vi "曲线对齐 - 副本.vi"() -> ()   [LabVIEW 2015]
uses:
  <vilib>/Utility/miscctls.llb/LVCursorListTypeDef.ctl
  <vilib>/Utility/file.llb/Read Delimited Spreadsheet (DBL).vi
panel:
  in  "确认修改":bool
  in  "功能选择":enum16{"无", "缩放实际曲线", "缩放理论曲线"}(ring)
  in  "加载数据":bool
  out "XY图 3":cluster{"理论时间":dbl[], "力":dbl[]}[](graph)
  out "all rows 2":dbl[][](array[numeric]) caption="所有行"
  in  "理论曲线路径":path=path "D:/曲线处理/理论1.csv" caption="理论"
  out "all rows":dbl[][](array[numeric]) caption="所有行"
  in  "测量曲线路径":path=path "D:/曲线处理/实测1.csv" caption="实际"
  in  "Enqueue Element":bool caption="元素入队列"
  in  "时间缩放 2":dbl=1.0
  in  "确定移动":bool
  out "输出簇 4":cluster{"x":dbl[], "y":dbl[]}
  out "输出簇 3":cluster{"x":dbl[], "y":dbl[]}
  out "输出簇 2":cluster{"x":dbl[], "y":dbl[]}
  out "输出簇1":cluster{"x":dbl[], "y":dbl[]}
  out "XY图 2":cluster{"x":dbl[], "y":dbl[]}[](graph)
  out "Position.X":dbl
  out "min(x,y)":dbl
  out "max(x,y)":dbl
  out "游标位置":cluster{"X":dbl, "Y":dbl}
  in  "动作":enum16{"设置范围", "设置峰值", "移动峰值"}(ring)
  in  "停止":bool
  in  "max":dbl=12.0 format="%#_13g"
  in  "min":dbl
  in  "力偏移":dbl
  in  "力缩放":dbl=1.0
  in  "时间偏移":dbl
  in  "时间缩放":dbl=1.0
  out "XY图":cluster{dbl[], dbl[]}[](graph)
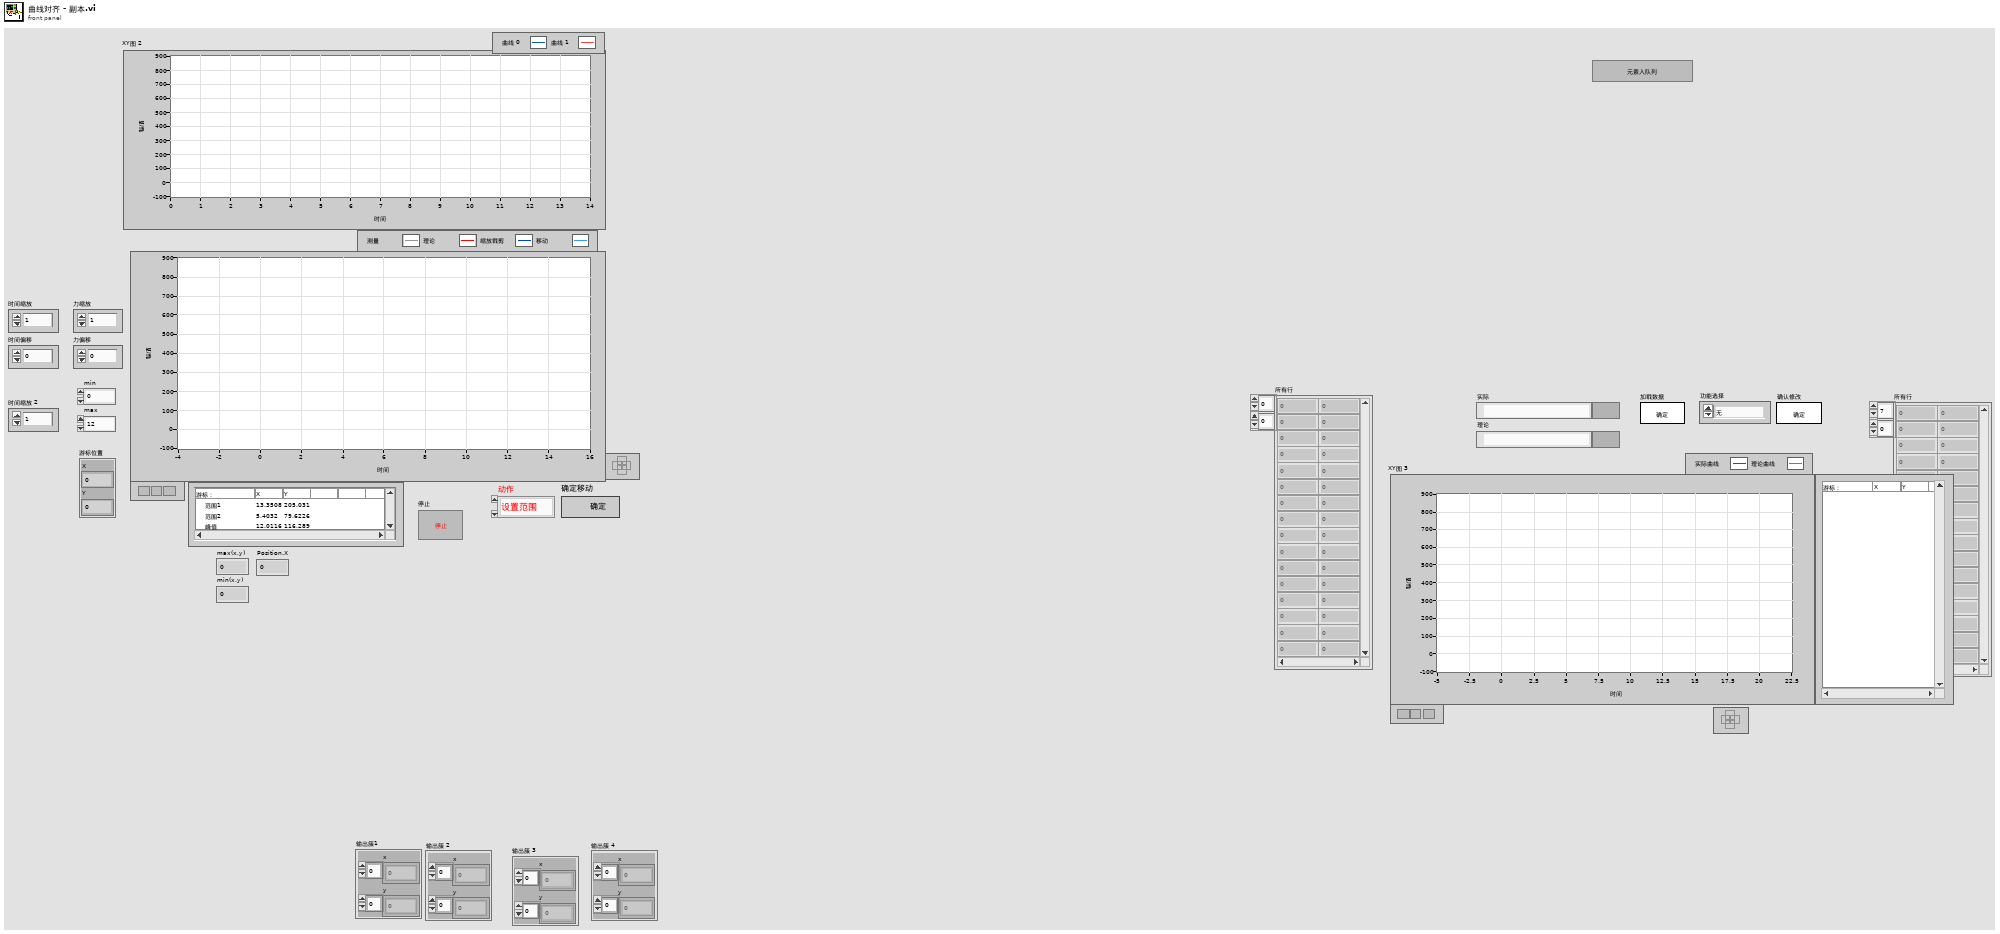
[diagram p1: front panel]
types:
  T1 = typedef "LVCursorListTypeDef.ctl" = cluster{"Name":string, "Color":u32, "Style":u8, "Point Style":u8, "Name Visible":bool, "Allow Drag":bool, "Cursor Mode":u32, "Plot":i32, "Index":i32, "Position":cluster{"X":dbl, "Y":dbl}, "X Scale":u32, "Y Scale":u32, "Watch Plots":i32[], "Watch All Plots":bool, "Plot Area":i32, "Label Offset":cluster{"X":dbl, "Y":dbl}}[]
  T2 = cluster{"Name":string, "Color":u32, "Style":u8, "Point Style":u8, "Name Visible":bool, "Allow Drag":bool, "Cursor Mode":u32, "Plot":i32, "Index":i32, "Position":cluster{"X":dbl, "Y":dbl}, "X Scale":u32, "Y Scale":u32, "Watch Plots":i32[], "Watch All Plots":bool, "Plot Area":i32, "Label Offset":cluster{"X":dbl, "Y":dbl}}
  T3 = cluster{"力":dbl[], "时间":dbl[], "理论力":dbl[], "理论时间":dbl[], "力预览":dbl[], "时间预览":dbl[]}
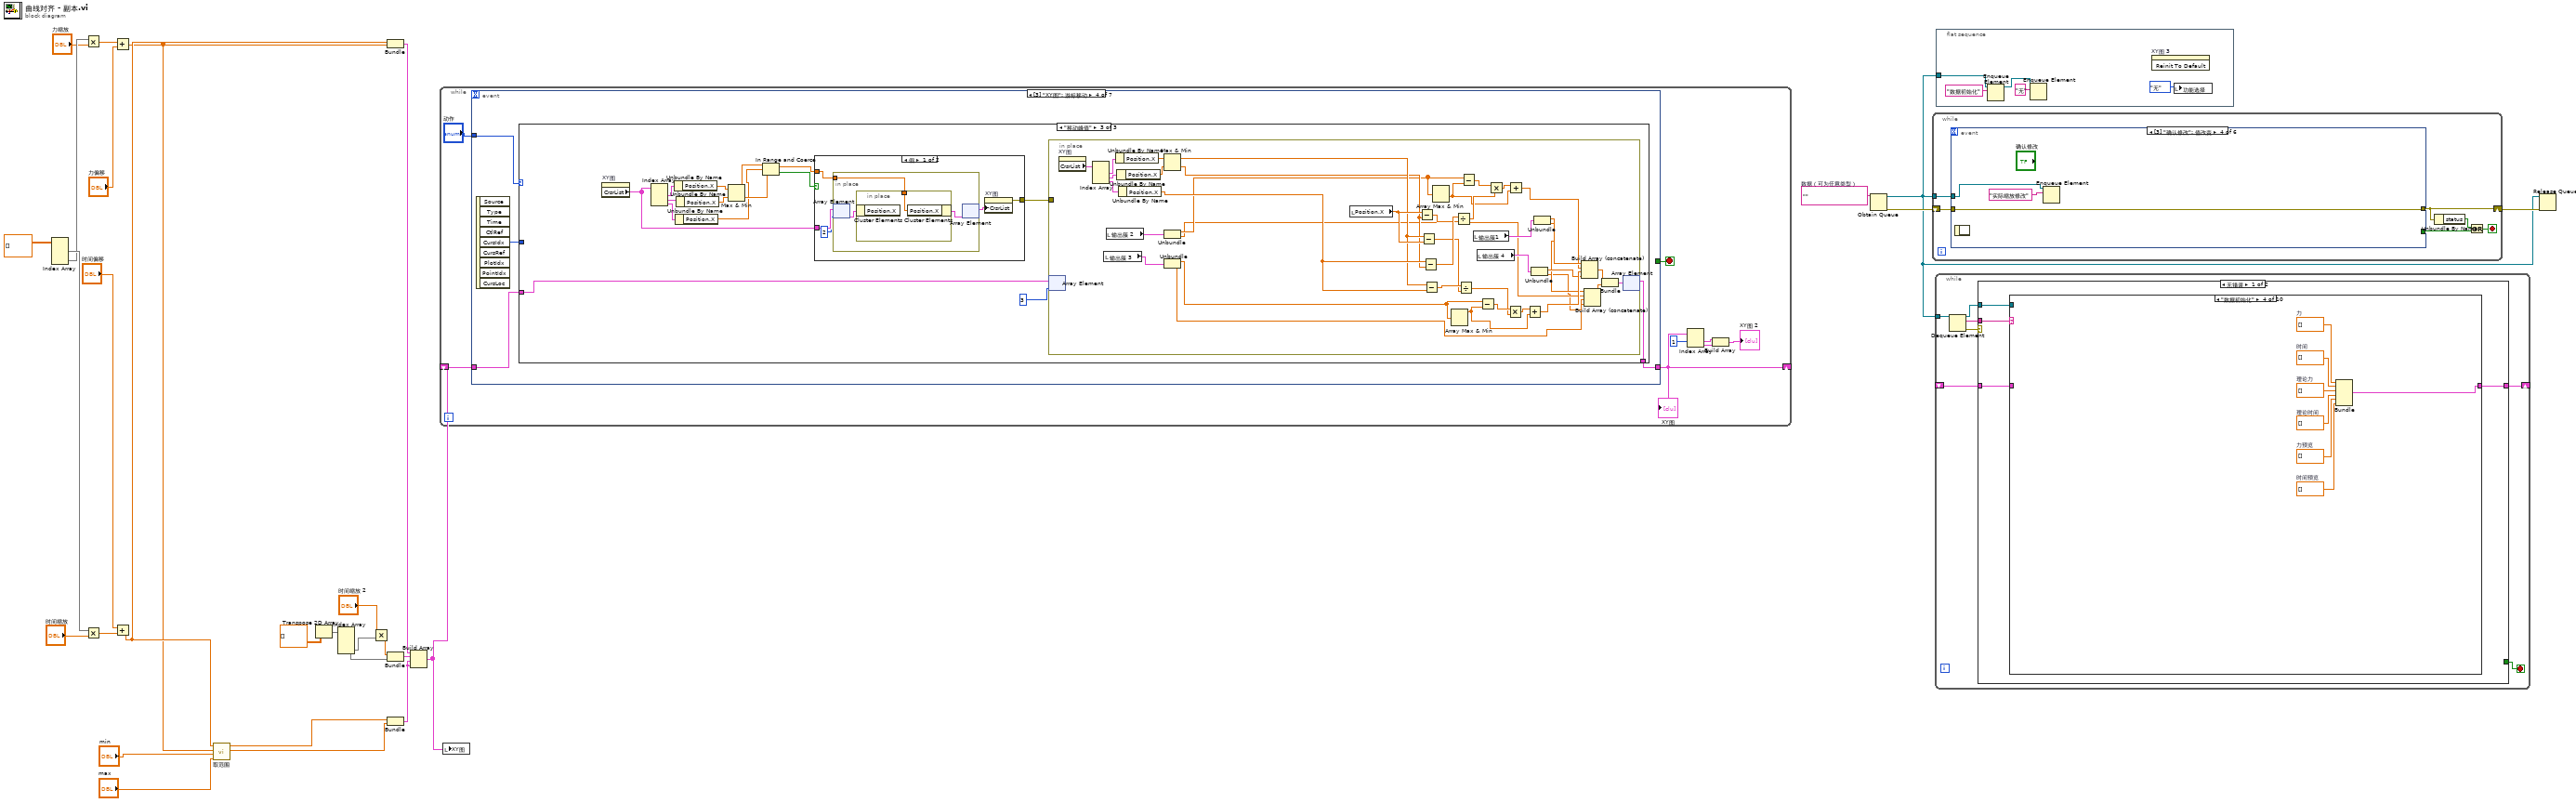
[diagram p0: block diagram]
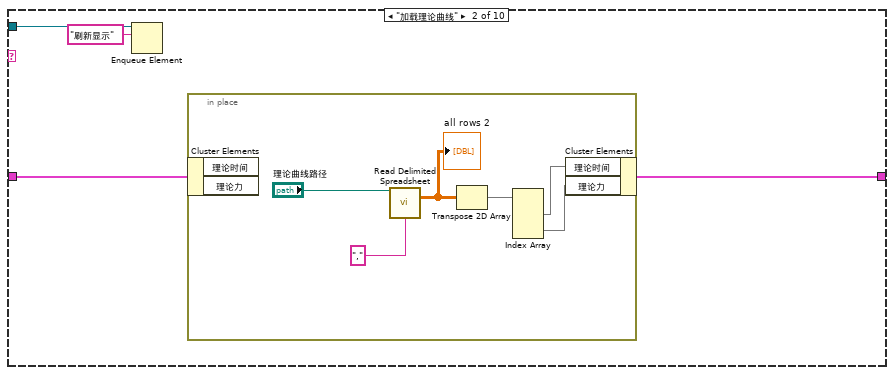
[diagram p3: hidden frame]
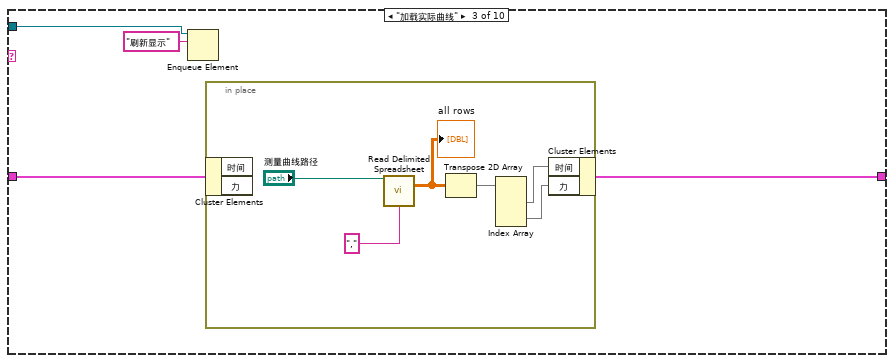
[diagram p4: hidden frame]
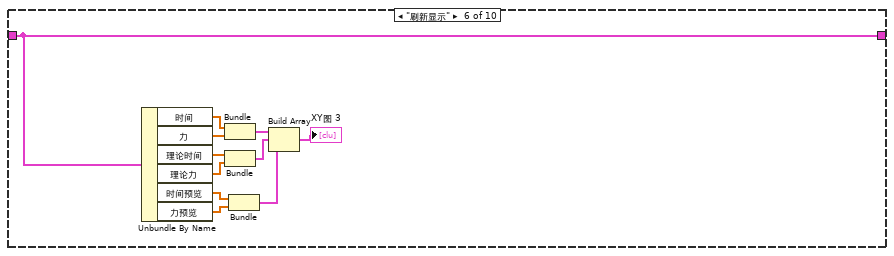
[diagram p6: hidden frame]
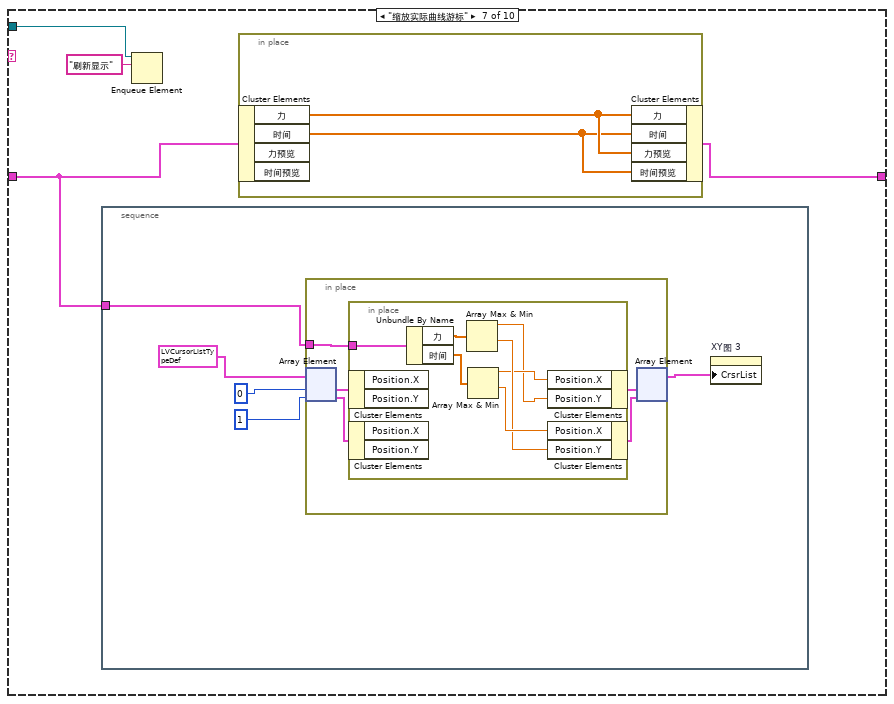
[diagram p7: hidden frame]
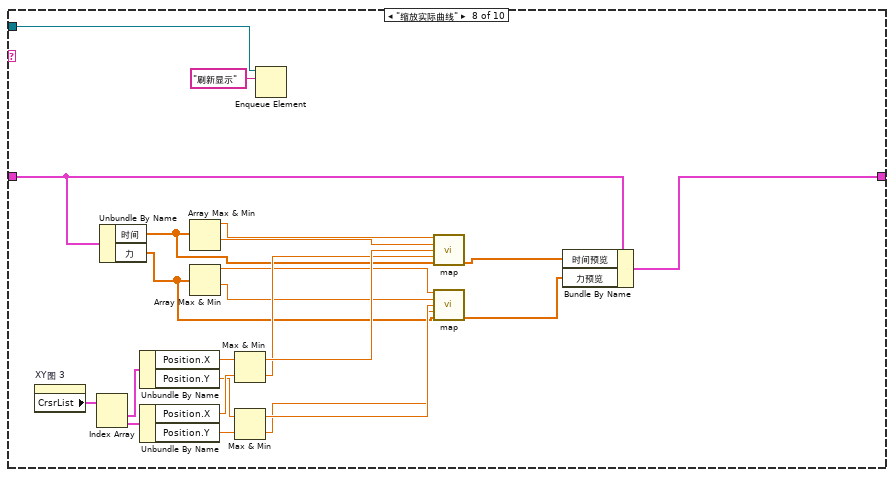
[diagram p8: hidden frame]
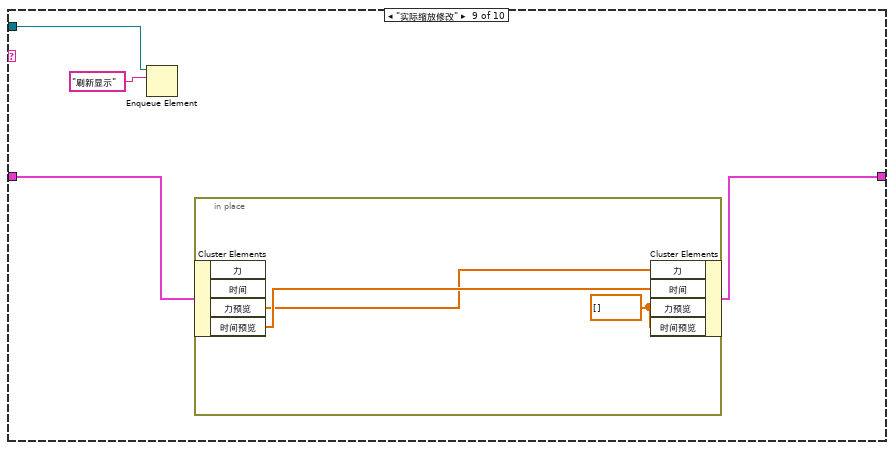
[diagram p9: hidden frame]
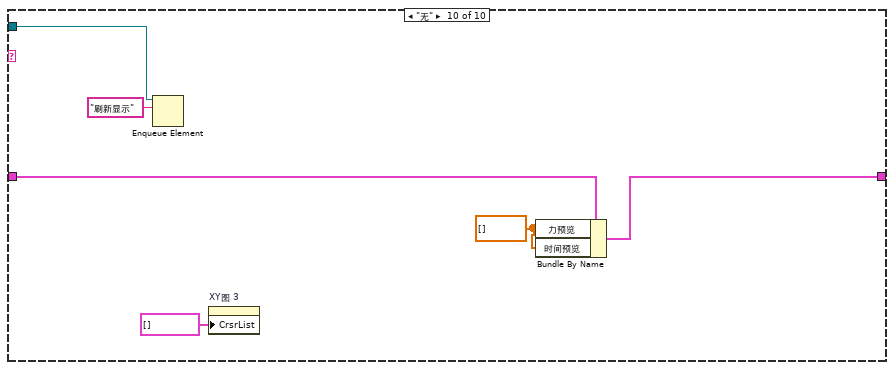
[diagram p10: hidden frame]
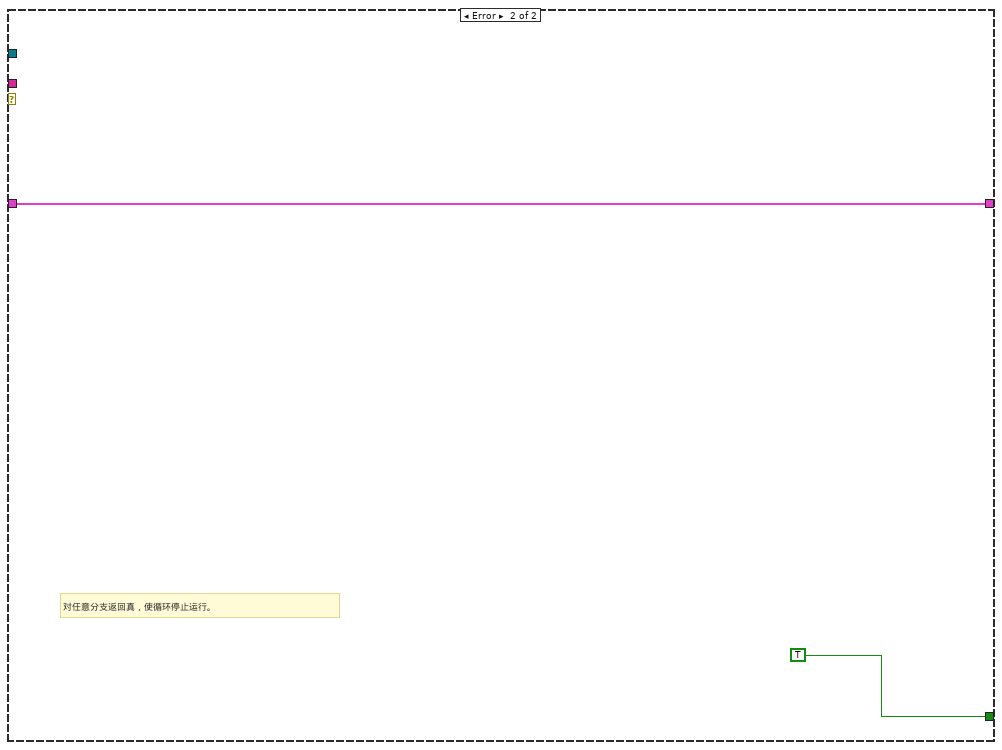
[diagram p11: hidden frame]
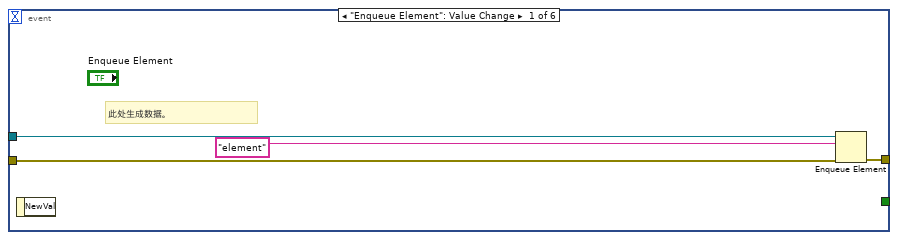
[diagram p12: hidden frame]
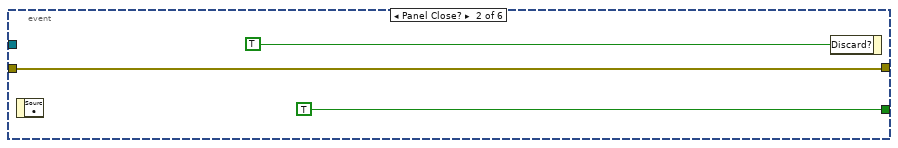
[diagram p13: hidden frame]
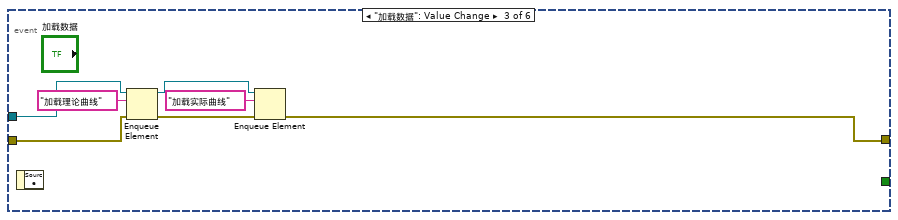
[diagram p14: hidden frame]
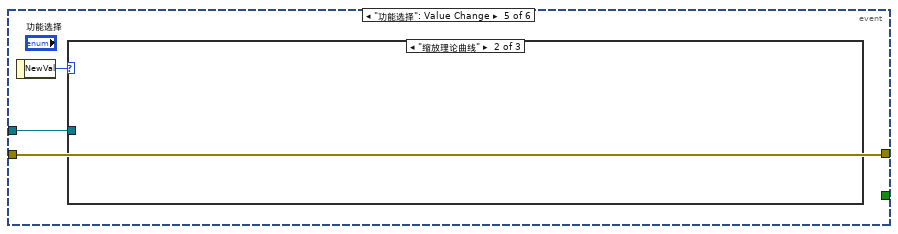
[diagram p15: hidden frame]
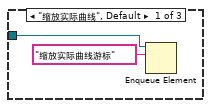
[diagram p16: hidden frame]
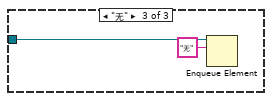
[diagram p17: hidden frame]
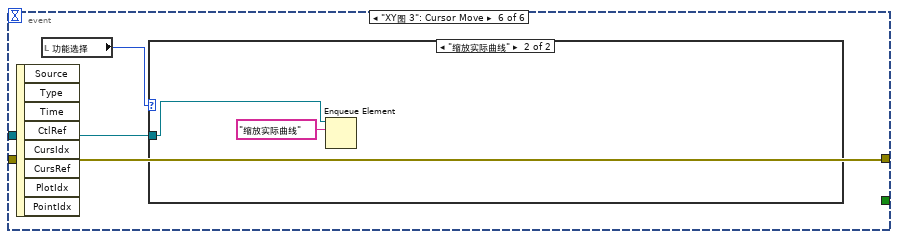
[diagram p18: hidden frame]
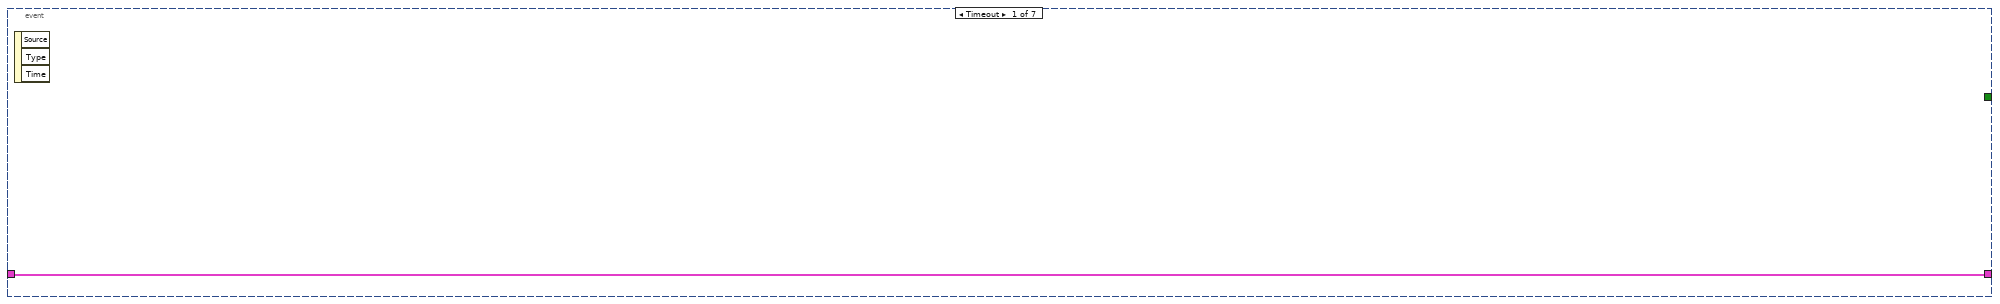
[diagram p20: hidden frame]
diagram:
  w6 = ""  # 数据（可为任意类型）
  n1 = Index Array(array=dbl[][] [] ("转置的数组")) -> (element #1=w25:dbl[], element #2=w21:dbl[])  [unwired: 4 in]
  n2 = Multiply(x=w21, y="力缩放") -> (x*y=w18:dbl[])
  n3 = Multiply(x=w25, y="时间缩放") -> (x*y=w22:dbl[])
  n4 = Add(x=w18, y="力偏移") -> (x+y=w12:dbl[])
  n5 = Add(x="时间偏移", y=w22) -> (x+y=w13:dbl[])
  n6 = call "取范围.vi"("max"="max", "min"="min", "y"=w12, "x"=w13) -> ("y"=w16:dbl[], "x"=w17:dbl[])  [unwired: 6 in]
  n7 = Transpose 2D Array(2D array=dbl[][] [] ("all rows")) -> (transposed array=w28:dbl[][])
  n8 = Index Array(array=w28) -> (element #1=w8:dbl[], element #2=w29:dbl[])  [unwired: 4 in]
  n9 = Multiply(x="时间缩放 2", y=w8) -> (x*y=w7:dbl[])
  n10 = Bundle(w13, w12) -> (w26:cluster{dbl[], dbl[]})  [unwired: 1 in]
  n11 = Bundle(w7, w29) -> (w27:cluster{dbl[], dbl[]})  [unwired: 1 in]
  n12 = Bundle("x"=w17, "y"=w16) -> (w11:cluster{"x":dbl[], "y":dbl[]})  [unwired: 1 in]
  n13 = Build Array(w26, w27, w11, w11) -> (w10:cluster{"x":dbl[], "y":dbl[]}[])
  n14 = while {
    shift-right: [w34] -> _
    shift-left: w10 -> [w35]
    stop <- w37 stop-if-true
    n15 = event shown="[3] \"XY图\": 游标移动" {
      selector: _ -> [_ _ _ _ _ _ _]
      dyn-events: _ -> [_ _ _ _ _ _ _]
      timeout: _ -> [_ _ _ _ _ _ _]
      tunnel: [_ _ _ _ _ _ TRUE] -> w37
      tunnel: "动作" -> [_ w40 w54 w66 _ _ _]
      tunnel: w35 -> [w38 w39 w53 w64 w163 w166 w211]
      tunnel: [w38 w39 w53 w63 w162 w166 w211] -> w34
      event Timeout {
        n16 = event-data() -> ()  [unwired: 1 in, 3 out]
      }
      event "XY图": event type 3.0.x80000027 {
        n17 = event-data() -> ("CursIdx"=w42:i32)  [unwired: 1 in, 7 out]
        n18 = case shown="\"设置峰值\"" w40 {
          tunnel: w42 -> [w45 w48 w51]
          tunnel: [w43 w46 w49] -> w41
          frame "设置范围", Default {
            n19 = Equal?(x=w45, y=2) -> (x = y?=w43:bool)
          }
          frame "设置峰值" {
            n20 = Not Equal?(x=w48, y=2) -> (x != y?=w46:bool)
          }
          frame "移动峰值" {
            n21 = Not Equal?(x=w51, y=2) -> (x != y?=w49:bool)
          }
        }
        n22 = event-data("Discard?"=w41) -> ()  [unwired: 1 in, 1 out]
      }
      event "XY图": Cursor Release {
        n23 = event-data() -> ("CursLoc"=→"游标位置":cluster{"X":dbl, "Y":dbl})  [unwired: 1 in, 8 out]
        n24 = property on="XY图" class="XYGraph (严格)"() -> ("CrsrList"=w52:T1)  [unwired: 2 in, 2 out]
        n25 = case shown="\"设置范围\", 默认" w54 {
          tunnel: w52 -> [w56 _ _]
          frame "设置范围", Default {
            n26 = Index Array(array=w56) -> (element #1=w62:T2, element #2=w61:T2)  [unwired: 2 in]
            n27 = Unbundle By Name(w62) -> ("Position.X"=w60:dbl)
            n28 = Unbundle By Name(w61) -> ("Position.X"=w59:dbl)
            n29 = Max & Min(x=w60, y=w59) -> (max(x,y)=→"max(x,y)":dbl, min(x,y)=→"min(x,y)":dbl)
          }
          frame "设置峰值" {
          }
          frame "移动峰值" {
          }
        }
      }
      event "XY图": Cursor Move {
        n30 = event-data() -> ("CursIdx"=w65:i32)  [unwired: 1 in, 8 out]
        n31 = case shown="\"移动峰值\"" w66 {
          tunnel: w65 -> [_ w76 _]
          tunnel: w64 -> [w67 w68 w112]
          tunnel: [w67 w68 w98] -> w63
          frame "设置范围", Default {
          }
          frame "设置峰值" {
            n32 = Equal?(x=w76, y=2) -> (x = y?=w74:bool)
            n33 = case shown="真" w74 {
              tunnel: [_ w77] -> w69
              frame False {
              }
              frame True {
                n34 = property on="XY图" class="XYGraph (严格)"() -> ("CrsrList"=w78:T1)  [unwired: 2 in, 2 out]
                n35 = Index Array(array=w78) -> (element #1=w87:T2, element #2=w86:T2, element #3=w88:T2)  [unwired: 3 in]
                n36 = Unbundle By Name(w87) -> ("Position.X"=w85:dbl)
                n37 = Unbundle By Name(w88) -> ("Position.X"=w81:dbl)
                n38 = Unbundle By Name(w86) -> ("Position.X"=w84:dbl)
                n39 = Max & Min(x=w85, y=w84) -> (max(x,y)=w83:dbl, min(x,y)=w82:dbl)
                n40 = In Range and Coerce(upper limit=w83, x=w81, lower limit=w82) -> (coerced(x)=w79:dbl, In Range?=w80:bool)
                n41 = case shown="假" w80 {
                  tunnel: w79 -> [w91 _]
                  tunnel: w78 -> [w93 _]
                  tunnel: [w89 _] -> w77
                  frame False {
                    n42 = in-place {
                      in-place-border: w91 -> [w95]
                      n43 = in-place-array #1(w93, 2) -> (w96:T2)
                      n44 = in-place {
                        in-place-border: w95 -> [w97]
                        n45 = in-place-cluster #2(w96) -> ()  [unwired: 1 out]
                        n46 = in-place-cluster #2("Position.X"=w97) -> (w94:T2)
                      }
                      n47 = in-place-array #1(w94) -> (w90:T1)  [unwired: 1 out]
                    }
                    n48 = property on="XY图" class="XYGraph (严格)"("CrsrList"=w90) -> (error out=w89:errorcluster)  [unwired: 2 in, 1 out]
                  }
                  frame True {
                  }
                }
              }
            }
            n49 = property on="XY图" class="XYGraph (严格)"(error in=w69) -> ("CrsrList"=w73:T1)  [unwired: 1 in, 2 out]
            n50 = Index Array(array=w73, index=2 ("索引")) -> (element=w71:T2)
            n51 = Unbundle By Name(w71) -> ("Position.X"=→"Position.X":dbl)
          }
          frame "移动峰值" {
            n52 = property on="XY图" class="XYGraph (严格)"() -> ("CrsrList"=w100:T1)  [unwired: 2 in, 2 out]
            n53 = Index Array(array=w100) -> (element #1=w109:T2, element #2=w108:T2, element #3=w110:T2)  [unwired: 3 in]
            n54 = Unbundle By Name(w109) -> ("Position.X"=w107:dbl)
            n55 = Unbundle By Name(w110) -> ("Position.X"=w103:dbl)
            n56 = Unbundle By Name(w108) -> ("Position.X"=w106:dbl)
            n57 = Max & Min(x=w107, y=w106) -> (max(x,y)=w105:dbl, min(x,y)=w104:dbl)
            n58 = In Range and Coerce(upper limit=w105, x=w103, lower limit=w104) -> (coerced(x)=w101:dbl, In Range?=w102:bool)
            n59 = case shown="假" w102 {
              tunnel: w101 -> [w115 _]
              tunnel: w100 -> [w117 _]
              tunnel: [w113 _] -> w99
              frame False {
                n60 = in-place {
                  in-place-border: w115 -> [w119]
                  n61 = in-place-array #3(w117, 2) -> (w120:T2)
                  n62 = in-place {
                    in-place-border: w119 -> [w121]
                    n63 = in-place-cluster #4(w120) -> ()  [unwired: 1 out]
                    n64 = in-place-cluster #4("Position.X"=w121) -> (w118:T2)
                  }
                  n65 = in-place-array #3(w118) -> (w114:T1)  [unwired: 1 out]
                }
                n66 = property on="XY图" class="XYGraph (严格)"("CrsrList"=w114) -> (error out=w113:errorcluster)  [unwired: 2 in, 1 out]
              }
              frame True {
              }
            }
            n67 = in-place {
              in-place-border: w99 -> [_]
              n68 = in-place-array #5(w112, 3) -> ()  [unwired: 1 out]
              n69 = property on="XY图" class="XYGraph (严格)"() -> ("CrsrList"=w160:T1)  [unwired: 2 in, 2 out]
              n70 = Index Array(array=w160) -> (element #1=w159:T2, element #2=w158:T2, element #3=w155:T2)  [unwired: 3 in]
              n71 = local read "输出簇 3"() -> (w138:cluster{"x":dbl[], "y":dbl[]})
              n72 = local read "输出簇 2"() -> (w139:cluster{"x":dbl[], "y":dbl[]})
              n73 = Unbundle By Name(w159) -> ("Position.X"=w157:dbl)
              n74 = Unbundle By Name(w158) -> ("Position.X"=w156:dbl)
              n75 = Unbundle By Name(w155) -> ("Position.X"=w153:dbl)
              n76 = Unbundle(w139) -> ("x"=w137:dbl[], "y"=w127:dbl[])
              n77 = Unbundle(w138) -> ("x"=w136:dbl[], "y"=w122:dbl[])
              n78 = Max & Min(x=w157, y=w156) -> (max(x,y)=w152:dbl, min(x,y)=w151:dbl)
              n79 = local read "Position.X"() -> (w154:dbl)
              n80 = Subtract(x=w154, y=w151) -> (x-y=w149:dbl)
              n81 = Subtract(x=w152, y=w154) -> (x-y=w147:dbl)
              n82 = Subtract(x=w153, y=w151) -> (x-y=w150:dbl)
              n83 = Subtract(x=w152, y=w153) -> (x-y=w148:dbl)
              n84 = Array Max & Min(array=w137) -> (min value=w143:dbl)  [unwired: 3 out]
              n85 = Array Max & Min(array=w136) -> (max value=w135:dbl)  [unwired: 3 out]
              n86 = Divide(x=w150, y=w149) -> (x/y=w145:dbl)
              n87 = Divide(x=w148, y=w147) -> (x/y=w140:dbl)
              n88 = Subtract(x=w137, y=w143) -> (x-y=w146:dbl[])
              n89 = local read "输出簇1"() -> (w134:cluster{"x":dbl[], "y":dbl[]})
              n90 = local read "输出簇 4"() -> (w133:cluster{"x":dbl[], "y":dbl[]})
              n91 = Subtract(x=w136, y=w135) -> (x-y=w141:dbl[])
              n92 = Multiply(x=w146, y=w145) -> (x*y=w144:dbl[])
              n93 = Multiply(x=w141, y=w140) -> (x*y=w142:dbl[])
              n94 = Add(x=w144, y=w143) -> (x+y=w131:dbl[])
              n95 = Add(x=w142, y=w135) -> (x+y=w130:dbl[])
              n96 = Unbundle(w133) -> ("x"=w129:dbl[], "y"=w126:dbl[])
              n97 = Unbundle(w134) -> ("x"=w132:dbl[], "y"=w128:dbl[])
              n98 = Build Array (concatenate)(w132, w131, w130, w129) -> (w125:dbl[])
              n99 = Build Array (concatenate)(w128, w127, w122, w126) -> (w124:dbl[])
              n100 = Bundle(w125, w124) -> (w123:cluster{dbl[], dbl[]})  [unwired: 1 in]
              n101 = in-place-array #5(w123) -> (w98:cluster{"x":dbl[], "y":dbl[]}[])  [unwired: 1 out]
            }
          }
        }
      }
      event "确定移动": Value Change {
        n102 = event-data() -> ()  [unwired: 1 in, 6 out]
        n103 = in-place {
          n104 = in-place-array #6(w163, 2, 3) -> (w165:cluster{"x":dbl[], "y":dbl[]})  [unwired: 1 out]
          n105 = in-place-array #6(w165, w165) -> (w162:cluster{"x":dbl[], "y":dbl[]}[])  [unwired: 2 out]
        }
      }
      event "动作": Value Change {
        n106 = event-data() -> ("NewVal"=w167:enum16{"设置范围", "设置峰值", "移动峰值"})  [unwired: 1 in, 5 out]
        n107 = case shown="\"设置峰值\"" w167 {
          tunnel: w166 -> [_ _ w189]
          frame "设置范围", Default {
          }
          frame "设置峰值" {
            n108 = case shown="真" TRUE {
              frame False {
              }
              frame True {
                n109 = property on="XY图" class="XYGraph (严格)"() -> ("CrsrList"=w176:T1)  [unwired: 2 in, 2 out]
                n110 = Index Array(array=w176) -> (element #1=w178:T2, element #2=w177:T2)  [unwired: 2 in]
                n111 = Unbundle By Name(w178) -> ("Position.X"=w175:dbl)
                n112 = Unbundle By Name(w177) -> ("Position.X"=w174:dbl)
                n113 = Add(x=w175, y=w174) -> (x+y=w173:dbl)
                n114 = Divide(x=w173, y=2.0) -> (x/y=w169:dbl)
                n115 = local write "Position.X"(w169) -> ()
                n116 = in-place {
                  in-place-border: w169 -> [w179]
                  n117 = in-place-array #7(w176, 2) -> (w181:T2)
                  n118 = in-place {
                    in-place-border: w179 -> [w182]
                    n119 = in-place-cluster #8(w181) -> ()  [unwired: 1 out]
                    n120 = in-place-cluster #8("Position.X"=w182) -> (w180:T2)
                  }
                  n121 = in-place-array #7(w180) -> (w170:T1)  [unwired: 1 out]
                }
                n122 = property on="XY图" class="XYGraph (严格)"("CrsrList"=w170) -> ()  [unwired: 2 in, 2 out]
              }
            }
          }
          frame "移动峰值" {
            n123 = Index Array(array=w189, index=2 ("索引")) -> (element=w187:cluster{"x":dbl[], "y":dbl[]})
            n124 = property on="XY图" class="XYGraph (严格)"() -> ("CrsrList"=w210:T1)  [unwired: 2 in, 2 out]
            n125 = Unbundle(w187) -> ("x"=w203:dbl[], "y"=w202:dbl[])
            n126 = Index Array(array=w210) -> (element #1=w209:T2, element #2=w208:T2, element #3=w205:T2)  [unwired: 3 in]
            n127 = Array Max & Min(array=w203) -> (max value=w201:dbl, min value=w204:dbl)  [unwired: 2 out]
            n128 = Unbundle By Name(w209) -> ("Position.X"=w207:dbl)
            n129 = Unbundle By Name(w208) -> ("Position.X"=w206:dbl)
            n130 = Unbundle By Name(w205) -> ("Position.X"=w196:dbl)
            n131 = Max & Min(x=w207, y=w206) -> (max(x,y)=w195:dbl, min(x,y)=w194:dbl)
            n132 = call "取范围.vi"("max"=w194, "min"=w204, "y"=w202, "x"=w203) -> ("y"=w199:dbl[], "x"=w200:dbl[])  [unwired: 6 in]
            n133 = call "取范围.vi"("max"=w196, "min"=w194, "y"=w202, "x"=w203) -> ("y"=w190:dbl[], "x"=w193:dbl[])  [unwired: 6 in]
            n134 = call "取范围.vi"("max"=w195, "min"=w196, "y"=w202, "x"=w203) -> ("y"=w191:dbl[], "x"=w192:dbl[])  [unwired: 6 in]
            n135 = call "取范围.vi"("max"=w201, "min"=w195, "y"=w202, "x"=w203) -> ("y"=w197:dbl[], "x"=w198:dbl[])  [unwired: 6 in]
            n136 = Bundle("x"=w200, "y"=w199) -> (→"输出簇1":cluster{"x":dbl[], "y":dbl[]})  [unwired: 1 in]
            n137 = Bundle("x"=w192, "y"=w191) -> (→"输出簇 3":cluster{"x":dbl[], "y":dbl[]})  [unwired: 1 in]
            n138 = Bundle("x"=w198, "y"=w197) -> (→"输出簇 4":cluster{"x":dbl[], "y":dbl[]})  [unwired: 1 in]
            n139 = Bundle("x"=w193, "y"=w190) -> (→"输出簇 2":cluster{"x":dbl[], "y":dbl[]})  [unwired: 1 in]
          }
        }
      }
      event "停止": Value Change {
        n140 = event-data() -> ()  [unwired: 1 in, 6 out]
      }
    }
    "XY图" <- w34
    n141 = Index Array(array=w34, index #1=1 ("索引")) -> (element #1=w32:cluster{"x":dbl[], "y":dbl[]}, element #2=w31:cluster{"x":dbl[], "y":dbl[]})  [unwired: 1 in]
    n142 = Build Array(w32, w31) -> (→"XY图 2":cluster{"x":dbl[], "y":dbl[]}[])
  }
  n143 = local write "XY图"(w10) -> ()
  n144 = Obtain Queue(element data type=w6) -> (queue out=w1:refnum<queue>, error out=w4:errorcluster)  [unwired: 4 in, 1 out]
  n145 = while {
    shift-right: [w214] -> w5
    shift-left: w4 -> [w217]
    tunnel: w1 -> [w218]
    stop <- w215 stop-if-true
    n146 = event shown="[3] \"确认修改\": 值改变" {
      selector: _ -> [_ _ _ _ _ _]
      dyn-events: _ -> [_ _ _ _ _ _]
      timeout: _ -> [_ _ _ _ _ _]
      tunnel: w218 -> [w222 _ w230 w233 w236 w243]
      tunnel: w217 -> [w221 w225 w227 w235 w238 w245]
      tunnel: [w220 w225 w226 w235 w238 w245] -> w214
      tunnel: [_ TRUE ("stop") _ _ _ _] -> w216
      event "Enqueue Element": Value Change {
        # "此处生成数据。"
        n147 = event-data() -> ()  [unwired: 1 in, 1 out]
        n148 = Enqueue Element(queue=w222, element="element", error in (no error)=w221) -> (error out=w220:errorcluster)  [unwired: 1 in, 2 out]
      }
      event Panel Close? {
        n149 = event-data() -> ()  [unwired: 1 in, 1 out]
        n150 = event-data("Discard?"=TRUE ("放弃？")) -> ()  [unwired: 1 in, 1 out]
      }
      event "加载数据": Value Change {
        n151 = event-data() -> ()  [unwired: 1 in, 1 out]
        n152 = Enqueue Element(queue=w230, element="加载理论曲线" ("元素"), error in (no error)=w227) -> (queue out=w229:refnum<queue>, error out=w228:errorcluster)  [unwired: 1 in, 1 out]
        n153 = Enqueue Element(queue=w229, element="加载实际曲线" ("元素"), error in (no error)=w228) -> (error out=w226:errorcluster)  [unwired: 1 in, 2 out]
      }
      event "确认修改": Value Change {
        n154 = event-data() -> ()  [unwired: 1 in, 1 out]
        n155 = Enqueue Element(queue=w233, element="实际缩放修改" ("元素")) -> ()  [unwired: 2 in, 3 out]
      }
      event "功能选择": Value Change {
        n156 = event-data() -> ("NewVal"=w237:enum16{"无", "缩放实际曲线", "缩放理论曲线"})  [unwired: 1 in]
        n157 = case shown="\"缩放理论曲线\"" w237 {
          tunnel: w236 -> [w239 _ w242]
          frame "缩放实际曲线", Default {
            n158 = Enqueue Element(queue=w239, element="缩放实际曲线游标" ("元素")) -> ()  [unwired: 2 in, 3 out]
          }
          frame "缩放理论曲线" {
          }
          frame "无" {
            n159 = Enqueue Element(queue=w242, element="无" ("元素")) -> ()  [unwired: 2 in, 3 out]
          }
        }
      }
      event "XY图 3": Cursor Move {
        n160 = event-data() -> ()  [unwired: 1 in, 8 out]
        n161 = local read "功能选择"() -> (w244:enum16{"无", "缩放实际曲线", "缩放理论曲线"})
        n162 = case shown="\"缩放实际曲线\"" w244 {
          tunnel: w243 -> [_ w246]
          frame "无", Default {
          }
          frame "缩放实际曲线" {
            n163 = Enqueue Element(queue=w246, element="缩放实际曲线" ("元素")) -> ()  [unwired: 2 in, 3 out]
          }
        }
      }
    }
    n164 = Unbundle By Name(w214) -> ("status"=w213:bool)
    n165 = Or(x=w213, y=w216) -> (x .or. y?=w215:bool)
  }
  n166 = while {
    tunnel: w1 -> [w249]
    shift-right: [w251] -> _
    shift-left: _ -> [w250]
    stop <- w252 stop-if-true
    n167 = Dequeue Element(queue=w249) -> (queue out=w248:refnum<queue>, element=w253:string, error out=w254:errorcluster)  [unwired: 2 in, 1 out]
    n168 = case shown="无错误" w254 {
      tunnel: w253 -> [w258 _]
      tunnel: [_ TRUE] -> w252
      tunnel: [w257 w358] -> w251
      tunnel: w250 -> [w256 w358]
      tunnel: w248 -> [w255 _]
      frame No Error {
        n169 = case shown="\"数据初始化\"" w258 {
          tunnel: [w259 w262 w272 w284 w287 w298 w301 w326 w347 w355] -> w257
          tunnel: w256 -> [w259 w263 w273 _ w287 w298 w302 w327 w348 w356]
          tunnel: w255 -> [_ w261 w270 _ _ _ w299 w322 w345 w352]
          frame "假", Default {
          }
          frame "加载理论曲线" {
            n170 = Enqueue Element(queue=w261, element="刷新显示" ("元素")) -> ()  [unwired: 2 in, 3 out]
            n171 = in-place {
              n172 = in-place-cluster #9(w263) -> ()  [unwired: 2 out]
              n173 = call-poly <vilib>:"Read Delimited Spreadsheet.vi"("file path (dialog if empty)"="理论曲线路径", "delimiter (\\t)"="," ("delimiter (\\t)")) -> ("all rows"=w266:dbl[][])  [unwired: 8 in, 5 out]
              "all rows 2" <- w266
              n174 = Transpose 2D Array(2D array=w266) -> (transposed array=w267:dbl[][])
              n175 = Index Array(array=w267) -> (element #1=w265:dbl[], element #2=w264:dbl[])  [unwired: 4 in]
              n176 = in-place-cluster #9("理论时间"=w265, "理论力"=w264) -> (w262:T3)
            }
          }
          frame "加载实际曲线" {
            n177 = Enqueue Element(queue=w270, element="刷新显示" ("元素")) -> ()  [unwired: 2 in, 3 out]
            n178 = in-place {
              n179 = in-place-cluster #10(w273) -> ()  [unwired: 2 out]
              n180 = call-poly <vilib>:"Read Delimited Spreadsheet.vi"("file path (dialog if empty)"="测量曲线路径", "delimiter (\\t)"="," ("delimiter (\\t)")) -> ("all rows"=w278:dbl[][])  [unwired: 8 in, 5 out]
              "all rows" <- w278
              n181 = Transpose 2D Array(2D array=w278) -> (transposed array=w279:dbl[][])
              n182 = Index Array(array=w279) -> (element #1=w275:dbl[], element #2=w274:dbl[])  [unwired: 4 in]
              n183 = in-place-cluster #10("时间"=w275, "力"=w274) -> (w272:T3)
            }
          }
          frame "数据初始化" {
            w280 = dbl[] []  # 时间预览
            w281 = dbl[] []  # 力预览
            w282 = dbl[] []  # 理论时间
            w283 = dbl[] []  # 理论力
            w285 = dbl[] []  # 时间
            w286 = dbl[] []  # 力
            n184 = Bundle("力"=w286, "时间"=w285, "理论力"=w283, "理论时间"=w282, "力预览"=w281, "时间预览"=w280) -> (w284:T3)  [unwired: 1 in]
          }
          frame "原始数据缩放" {
          }
          frame "刷新显示" {
            n185 = Unbundle By Name(w298) -> ("时间"=w292:dbl[], "力"=w291:dbl[], "理论时间"=w297:dbl[], "理论力"=w296:dbl[], "时间预览"=w289:dbl[], "力预览"=w290:dbl[])
            n186 = Bundle("时间"=w292, "力"=w291) -> (w295:cluster{"时间":dbl[], "力":dbl[]})  [unwired: 1 in]
            n187 = Bundle("理论时间"=w297, "理论力"=w296) -> (w294:cluster{"理论时间":dbl[], "理论力":dbl[]})  [unwired: 1 in]
            n188 = Bundle("时间预览"=w289, "力预览"=w290) -> (w288:cluster{"时间预览":dbl[], "力预览":dbl[]})  [unwired: 1 in]
            n189 = Build Array(w295, w294, w288) -> (→"XY图 3":cluster{"时间预览":dbl[], "力预览":dbl[]}[])
          }
          frame "缩放实际曲线游标" {
            n190 = stacked-sequence {
              tunnel: w302 -> [w306]
              frame #0 {
                n191 = in-place {
                  in-place-border: w306 -> [w312]
                  n192 = in-place-array #11(T1 [{"Name"="游标0", "Color"=16711680, "Style"=8, "Point Style"=13, "Name Visible"=FALSE, "Allow Drag"=TRUE, "Cursor Mode"=0, "Plot"=0, "Index"=0, "Position"={"X"=24.900169204737733, "Y"=876.3513513513514}, "X Scale"=0, "Y Scale"=0, "Watch Plots"=[], "Watch All Plots"=FALSE, "Plot Area"=0, "Label Offset"={"X"=0.0, "Y"=67.56756756756761}}, {"Name"="游标1", "Color"=16860, "Style"=8, "Point Style"=13, "Name Visible"=FALSE, "Allow Drag"=TRUE, "Cursor Mode"=0, "Plot"=0, "Index"=0, "Position"={"X"=-2.199661590524536, "Y"=1.3513513513513553}, "X Scale"=0, "Y Scale"=0, "Watch Plots"=[], "Watch All Plots"=FALSE, "Plot Area"=0, "Label Offset"={"X"=8.881784197001252e-16, "Y"=67.56756756756756}}] ("游标列表"), 0, 1) -> (w314:T2, w313:T2)
                  n193 = in-place {
                    in-place-border: w312 -> [w319]
                    n194 = in-place-cluster #12(w314) -> ()  [unwired: 2 out]
                    n195 = in-place-cluster #13(w313) -> ()  [unwired: 2 out]
                    n196 = Unbundle By Name(w319) -> ("力"=w320:dbl[], "时间"=w321:dbl[])
                    n197 = Array Max & Min(array=w320) -> (max value=w315:dbl, min value=w317:dbl)  [unwired: 2 out]
                    n198 = Array Max & Min(array=w321) -> (max value=w316:dbl, min value=w318:dbl)  [unwired: 2 out]
                    n199 = in-place-cluster #12("Position.X"=w316, "Position.Y"=w315) -> (w311:T2)
                    n200 = in-place-cluster #13("Position.X"=w318, "Position.Y"=w317) -> (w310:T2)
                  }
                  n201 = in-place-array #11(w311, w310) -> (w305:T1)  [unwired: 2 out]
                }
                n202 = property on="XY图 3" class="XYGraph (严格)"("CrsrList"=w305) -> ()  [unwired: 2 in, 2 out]
              }
            }
            n203 = Enqueue Element(queue=w299, element="刷新显示" ("元素")) -> ()  [unwired: 2 in, 3 out]
            n204 = in-place {
              n205 = in-place-cluster #14(w302) -> ("力"=w304:dbl[], "时间"=w303:dbl[])  [unwired: 2 out]
              n206 = in-place-cluster #14("力"=w304, "时间"=w303, "力预览"=w304, "时间预览"=w303) -> (w301:T3)
            }
          }
          frame "缩放实际曲线" {
            n207 = property on="XY图 3" class="XYGraph (严格)"() -> ("CrsrList"=w344:T1)  [unwired: 2 in, 2 out]
            n208 = Index Array(array=w344) -> (element #1=w343:T2, element #2=w342:T2)  [unwired: 2 in]
            n209 = Unbundle By Name(w327) -> ("时间"=w333:dbl[], "力"=w328:dbl[])
            n210 = Unbundle By Name(w343) -> ("Position.X"=w341:dbl, "Position.Y"=w339:dbl)
            n211 = Unbundle By Name(w342) -> ("Position.X"=w340:dbl, "Position.Y"=w338:dbl)
            n212 = Array Max & Min(array=w333) -> (max value=w337:dbl, min value=w336:dbl)  [unwired: 2 out]
            n213 = Array Max & Min(array=w328) -> (max value=w332:dbl, min value=w331:dbl)  [unwired: 2 out]
            n214 = Max & Min(x=w341, y=w340) -> (max(x,y)=w335:dbl, min(x,y)=w334:dbl)
            n215 = Max & Min(x=w339, y=w338) -> (max(x,y)=w330:dbl, min(x,y)=w329:dbl)
            n216 = Enqueue Element(queue=w322, element="刷新显示" ("元素")) -> ()  [unwired: 2 in, 3 out]
            n217 = call "map.vi"("inmax"=w337, "inmin"=w336, "outmax"=w335, "outmin"=w334, "in"=w333) -> ("out"=w325:dbl[])  [unwired: 10 in]
            n218 = call "map.vi"("inmax"=w332, "inmin"=w331, "outmax"=w330, "outmin"=w329, "in"=w328) -> ("out"=w324:dbl[])  [unwired: 10 in]
            n219 = Bundle By Name(cluster=w327, "时间预览"=w325, "力预览"=w324) -> (w326:T3)
          }
          frame "实际缩放修改" {
            n220 = Enqueue Element(queue=w345, element="刷新显示" ("元素")) -> ()  [unwired: 2 in, 3 out]
            n221 = in-place {
              w349 = dbl[] [] ("力预览")
              n222 = in-place-cluster #15(w348) -> ("力预览"=w350:dbl[], "时间预览"=w351:dbl[])  [unwired: 2 out]
              n223 = in-place-cluster #15("力"=w350, "时间"=w351, "力预览"=w349, "时间预览"=w349) -> (w347:T3)
            }
          }
          frame "无" {
            w354 = dbl[] [] ("力预览")
            n224 = Enqueue Element(queue=w352, element="刷新显示" ("元素")) -> ()  [unwired: 2 in, 3 out]
            n225 = property on="XY图 3" class="XYGraph (严格)"("CrsrList"=T1 [] ("游标列表")) -> ()  [unwired: 2 in, 2 out]
            n226 = Bundle By Name(cluster=w356, "力预览"=w354, "时间预览"=w354) -> (w355:T3)
          }
        }
      }
      frame Error {
        # "对任意分支返回真，使循环停止运行。"
      }
    }
  }
  n227 = flat-sequence {
    tunnel: w1 -> [w363]
    frame #0 {
      n228 = Enqueue Element(queue=w363, element="数据初始化" ("元素")) -> (queue out=w360:refnum<queue>)  [unwired: 2 in, 2 out]
      n229 = Enqueue Element(queue=w360, element="无" ("元素")) -> ()  [unwired: 2 in, 3 out]
      n230 = invoke on="XY图 3" class="XYGraph (严格)" method="Reinit To Default"() -> ()  [unwired: 3 in, 3 out]
      n231 = local write "功能选择"(enum16{"无", "缩放实际曲线", "缩放理论曲线"}."无" ("功能选择")) -> ()
    }
  }
  n232 = Release Queue(queue=w1, error in (no error)=w5) -> ()  [unwired: 1 in, 3 out]
